vi "ReadValuesOfMoreTransmitters_VISA.vi"() -> ()   [LabVIEW 2012]
uses:
  utility/K_S30_VISA Global.vi
panel:
  in  "Time [ms]":u32=10
  in  "clear Log":bool
  in  "Start / Stop":bool
  in  "Stop":bool
  in  "Log":string
  out "values":sgl[](array[numeric])
  out "communication":bool[](array[boolean])
  out "error out":errorcluster
  in  "Devices":T1(array[cluster])=[{"Address"=1, "Channel"=enum."P1"}, {"Address"=2, "Channel"=enum."P1"}, {"Address"=2, "Channel"=enum."TOB1"}]
  # "simple demonstation how to read out values from n devices"
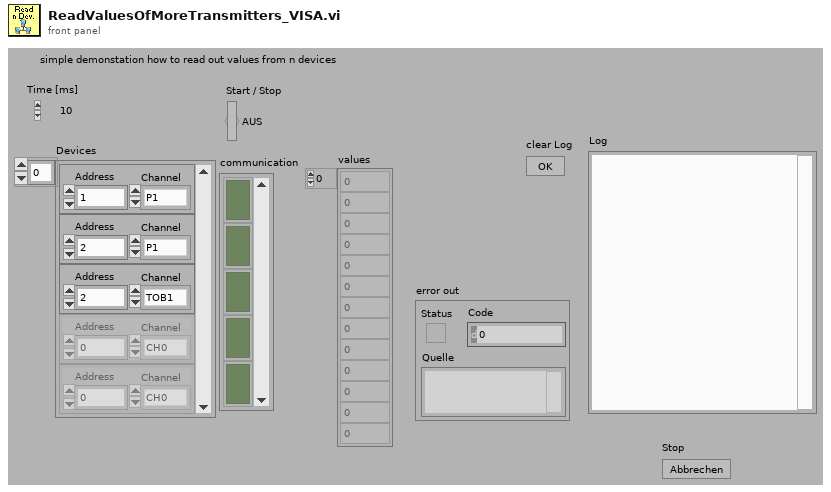
[diagram p1: front panel]
types:
  T1 = cluster{"Address":u8, "Channel":enum16{"CH0", "P1", "P2", "T", "TOB1", "TOB2"}}[]
  T2 = cluster{"Baudrate":enum16{"9600", "115200"}, "Echo":bool, "Timeout":u32, "VISA":refnum<visa-resource-name>}
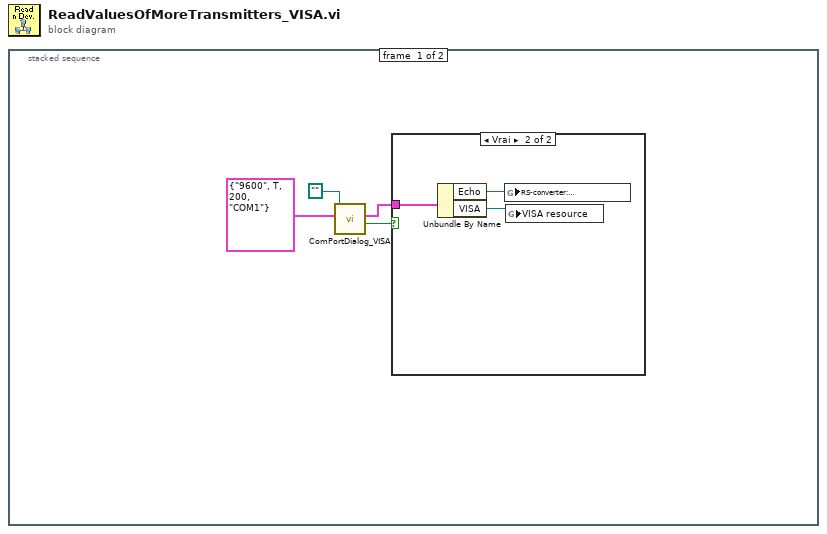
[diagram p0: block diagram]
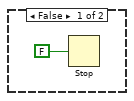
[diagram p2: hidden frame]
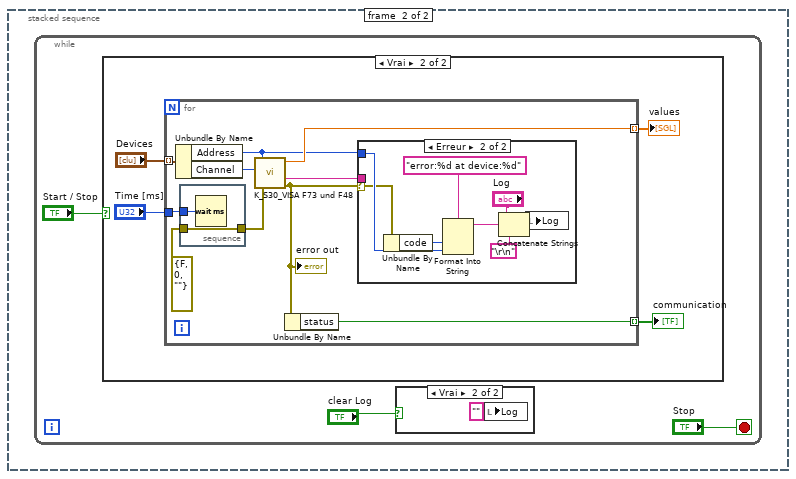
[diagram p3: hidden frame]
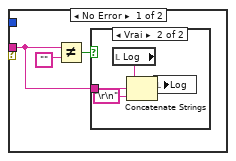
[diagram p6: hidden frame]
diagram:
  n1 = stacked-sequence {
    frame #0 {
      n2 = call "ComPortDialog_VISA.vi"("Com-Einst. in"=T2 {"Baudrate"=enum."9600", "Echo"=TRUE, "Timeout"=200, "VISA"="COM1"}, "ini-File"=path "") -> ("Abbruch"=w2:bool, "Com-Einst. out"=w1:T2)  [unwired: 8 in]
      n3 = case shown="Vrai" w2 {
        tunnel: w1 -> [_ w8]
        frame False {
          n4 = Stop(stop? (T)=FALSE ("Stop? (T)")) -> ()
        }
        frame True {
          n5 = Unbundle By Name(w8) -> ("Echo"=w6:bool, "VISA"=w7:refnum<visa-resource-name>)
          n6 = global write "K_S30_VISA Global.vi" "RS-converter:\necho"(w6) -> ()
          n7 = global write "K_S30_VISA Global.vi" "VISA resource"(w7) -> ()
        }
      }
    }
    frame #1 {
      n8 = while {
        stop <- "Stop" stop-if-true
        n9 = case shown="Vrai" "Start / Stop" {
          frame False {
          }
          frame True {
            n10 = for {
              tunnel: "Devices" -> [w26] mode=indexing
              tunnel: [w24] -> w15 mode=indexing
              tunnel: [w25] -> w14 mode=indexing
              tunnel: "Time [ms]" -> [w20]
              n11 = Unbundle By Name(w26) -> ("Address"=w23:u8, "Channel"=w22:enum16{"CH0", "P1", "P2", "T", "TOB1", "TOB2"})
              n12 = stacked-sequence {
                tunnel: w20 -> [w28]
                tunnel: [w27] -> w18
                tunnel: errorcluster {"status"=FALSE, "code"=0, "source"=""} ("error in (no error)") -> [w27]
                frame #0 {
                  n13 = Wait (ms)(milliseconds to wait=w28) -> ()  [unwired: 1 out]
                }
              }
              n14 = call "K_S30_VISA F73 und F48.vi"("error in"=w18, "Channel"=w22, "Address"=w23) -> ("error out"=w21:errorcluster, "msg"=w17:string, "Value"=w24:sgl)  [unwired: 1 in, 1 out]
              "error out" <- w21
              n15 = Unbundle By Name(w21) -> ("status"=w25:bool)
              n16 = case shown="Erreur" w21 {
                selector: w21 -> [_ w41]
                tunnel: w23 -> [_ w43]
                tunnel: w17 -> [w29 _]
                frame No Error {
                  n17 = Not Equal?(x=w29, y="") -> (x != y?=w30:bool)
                  n18 = case shown="Vrai" w30 {
                    tunnel: w29 -> [_ w32]
                    frame False {
                    }
                    frame True {
                      n19 = local read "Log"() -> (w35:string)
                      n20 = Concatenate Strings(w35, w32, "\r\n") -> (w34:string)
                      n21 = local write "Log"(w34) -> ()
                    }
                  }
                }
                frame Error {
                  n22 = Unbundle By Name(w41) -> ("code"=w40:i32)
                  n23 = Format Into String(format string="error:%d at device:%d" ("Format-String"), w40, w43) -> (resulting string=w36:string)  [unwired: 2 in, 1 out]
                  n24 = Concatenate Strings("Log", w36, "\r\n") -> (w38:string)
                  n25 = local write "Log"(w38) -> ()
                }
              }
            }
            "communication" <- w14
            "values" <- w15
          }
        }
        n26 = case shown="Vrai" "clear Log" {
          frame False {
          }
          frame True {
            n27 = local write "Log"("" ("Log")) -> ()
          }
        }
      }
    }
  }
